vi "ELL9 Send Command.vi"(0 "VISA Ref":refnum<visa-resource-name>, 2 "Wait for Reply (T)":bool=TRUE, 7 "Command":string, 11 "Error In":errorcluster) -> (4 "VISA Ref Dup":refnum<visa-resource-name>, 8 "Reply":string, 13 "Cmd Success":bool, 15 "Error Out":errorcluster)   [LabVIEW 2020]
uses:
  <vilib>/Utility/error.llb/whitespace.ctl
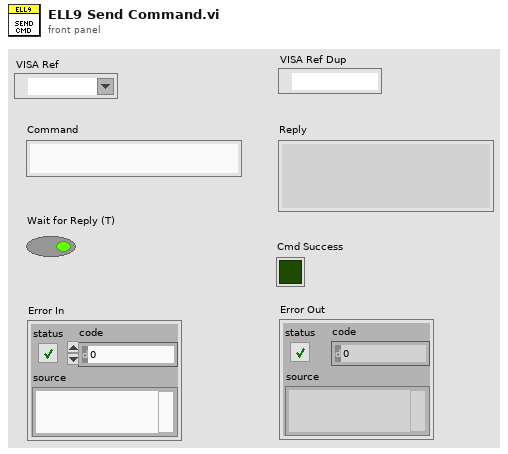
[diagram p1: front panel]
types:
  T1 = typedef "whitespace.ctl" = u16
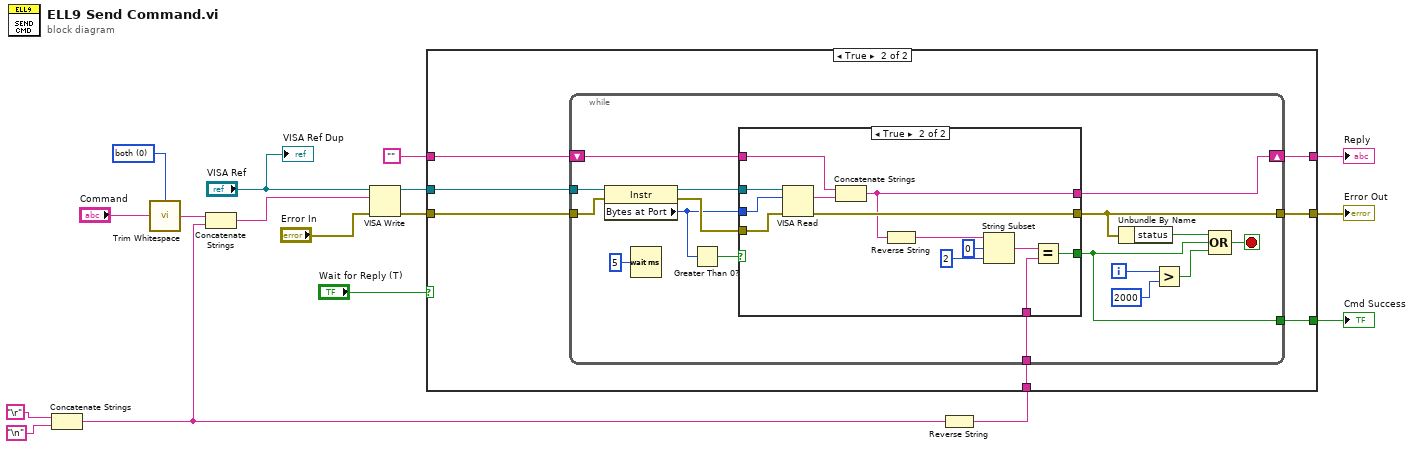
[diagram p0: block diagram]
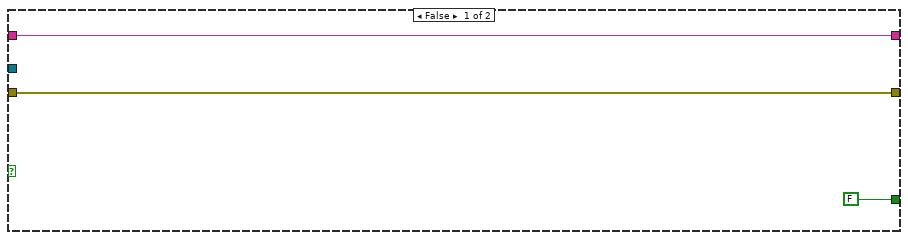
[diagram p2: hidden frame]
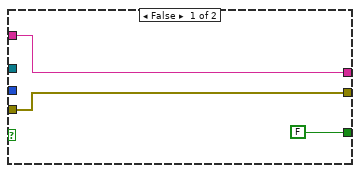
[diagram p3: hidden frame]
diagram:
  w16 = T1 0 items=["both", "start of string", "end of string"] ("location (both)")
  n1 = Concatenate Strings("\r", "\n") -> (w2:string)
  n2 = call <vilib>:"Trim Whitespace.vi"("string"="Command", "location (both)"=w16) -> ("trimmed string"=w15:string)
  n3 = Concatenate Strings(w15, w2) -> (w14:string)
  n4 = VISA Write(VISA resource name="VISA Ref", write buffer=w14, error in (no error)="Error In") -> (VISA resource name out=w13:refnum<visa-resource-name>, error out=w12:errorcluster)  [unwired: 1 out]
  n5 = Reverse String(1:w2) -> (0:w1:string)
  n6 = case shown="True" "Wait for Reply (T)" {
    tunnel: w13 -> [_ w23]
    tunnel: w12 -> [w20 w22]
    tunnel: "" -> [w19 w27]
    tunnel: [w19 w26] -> w6
    tunnel: [w20 w25] -> w8
    tunnel: w1 -> [_ w24]
    tunnel: [FALSE w21] -> w5
    frame False {
    }
    frame True {
      n7 = while {
        tunnel: w23 -> [w44]
        tunnel: w22 -> [w43]
        shift-right: [w32] -> w26
        shift-left: w27 -> [w33]
        tunnel: [w30] -> w25
        tunnel: w24 -> [w29]
        tunnel: [w28] -> w21
        i -> [w42]
        stop <- w39 stop-if-true
        n8 = property class="Instr"(reference=w44, error in=w43) -> (reference out=w35:refnum<visa-resource-name>, error out=w36:errorcluster, "Bytes at Port"=w34:u32)
        n9 = Wait (ms)(milliseconds to wait=u32 5) -> ()  [unwired: 1 out]
        n10 = Greater Than 0?(x=w34) -> (x > 0?=w37:bool)
        n11 = case shown="True" w37 {
          tunnel: w36 -> [w47 w59]
          tunnel: w35 -> [_ w60]
          tunnel: w34 -> [_ w58]
          tunnel: w33 -> [w45 w57]
          tunnel: [w45 w54] -> w32
          tunnel: [w47 w55] -> w30
          tunnel: [FALSE w50] -> w28
          tunnel: w29 -> [_ w49]
          frame False {
          }
          frame True {
            n12 = VISA Read(VISA resource name=w60, byte count=w58, error in (no error)=w59) -> (read buffer=w56:string, error out=w55:errorcluster)  [unwired: 2 out]
            n13 = Concatenate Strings(w57, w56) -> (w54:string)
            n14 = Reverse String(1:w54) -> (0:w48:string)
            n15 = String Subset(string=w48, offset (0)=0, length (rest)=2 ("length (rest)")) -> (substring=w51:string)
            n16 = Equal?(x=w51, y=w49) -> (x = y?=w50:bool)
          }
        }
        n17 = Unbundle By Name(w30) -> ("status"=w31:bool)
        n18 = Greater?(x=w42, y=2000) -> (0:w40:bool)
        n19 = Compound Arithmetic op=OR(w31, w28, w40) -> (w39:bool)
      }
    }
  }
  "Reply" <- w6
  "Error Out" <- w8
  "Cmd Success" <- w5
  "VISA Ref Dup" <- "VISA Ref"
